vi "Parse Metadata.vi"(11 "String":string) -> (3 "Metadata":T1[](array[typedef]))   [LabVIEW 2015, in "NI_Azure_Queue.lvlib"]
uses:
  NI_Azure_Queue.lvlib
  Core/Name Value Pair.ctl
  Core/NI_Azure_Core.lvlib
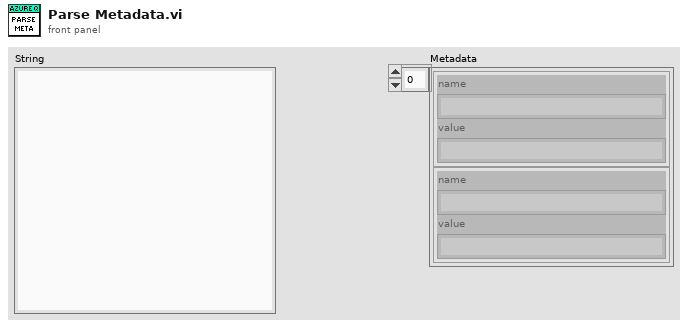
[diagram p1: front panel]
types:
  T1 = typedef "NI_Azure_Core.lvlib/Name Value Pair.ctl" = cluster{"name":string, "value":string}
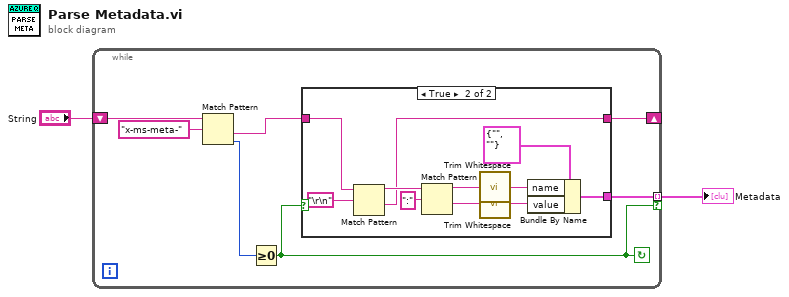
[diagram p0: block diagram]
diagram:
  n1 = while {
    shift-right: [w5] -> _
    shift-left: "String" -> [w9]
    tunnel: [w4] -> w1 mode=indexing if=w3
    stop <- w3 continue-if-true
    n2 = Match Pattern(string=w9, regular expression="x-ms-meta-") -> (after substring=w6:string, offset past match=w7:i32)  [unwired: 1 in, 2 out]
    n3 = Greater Or Equal To 0?(x=w7) -> (x >= 0?=w3:bool)
    n4 = case shown="True" w3 {
      tunnel: w6 -> [w10 w21]
      tunnel: [w10 w17] -> w5
      tunnel: [_ w13] -> w4
      frame False {
      }
      frame True {
        n5 = Match Pattern(string=w21, regular expression="\r\n") -> (before substring=w19:string, after substring=w17:string)  [unwired: 1 in, 2 out]
        n6 = Match Pattern(string=w19, regular expression=":") -> (before substring=w15:string, after substring=w14:string)  [unwired: 1 in, 2 out]
        n7 = call <vilib>:"Trim Whitespace.vi"("string"=w15) -> ("trimmed string"=w12:string)  [unwired: 1 in]
        n8 = call <vilib>:"Trim Whitespace.vi"("string"=w14) -> ("trimmed string"=w11:string)  [unwired: 1 in]
        n9 = Bundle By Name(cluster=T1 {"name"="", "value"=""} ("Cluster"), "name"=w12, "value"=w11) -> (w13:T1)
      }
    }
  }
  "Metadata" <- w1
